vi "DAQ_Power.vi"(9 "stop":bool) -> ()   [LabVIEW 2020]
uses:
  <vilib>/Utility/error.llb/DialogType.ctl
  <vilib>/ULx/Create Channel.llb/ULx Create Channel (AI-Voltage-Basic).vi
  <vilib>/ULx/Timing.llb/ULx Timing (Sample Clock).vi
  <vilib>/ULx/Read.llb/ULx Read (Analog Wfm 1Chan NSamp).vi
panel:
  out "Power Graph":waveform(dbl)(graph)
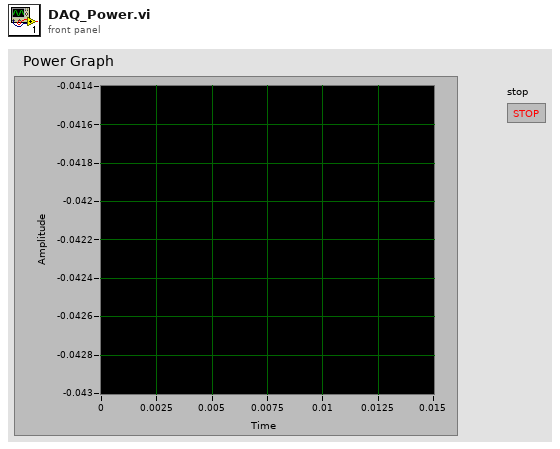
[diagram p1: front panel]
types:
  T1 = typedef "DialogType.ctl" = u16
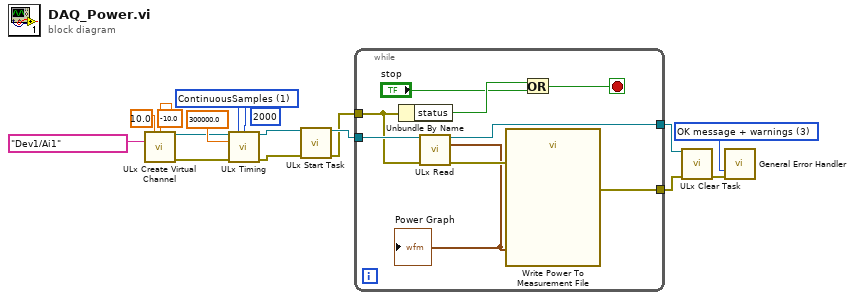
[diagram p0: block diagram]
diagram:
  w12 = 1 items=["FiniteSamples", "ContinuousSamples"] ("sample mode")
  w9 = T1 3 items=["no dialog", "OK message", "continue or stop message", "OK message + warnings", "continue/stop + warnings"] ("type of dialog (OK msg:1)")
  n1 = call-poly <vilib>:"ULx Create Virtual Channel.vi"("maximum value"=10.0, "minimum value"=-10.0, "physical channels"="Dev1/Ai1") -> ("task out"=w5:refnum<k24>, "error out"=w2:errorcluster)  [unwired: 11 in]
  n2 = call-poly <vilib>:"ULx Timing.vi"("task in"=w5, "sample mode"=w12, "samples per channel"=2000, "rate"=300000.0, "error in"=w2) -> ("task out"=w10:refnum<k24>, "error out"=w11:errorcluster)  [unwired: 9 in]
  n3 = call <vilib>:"ULx Start Task.vi"("task in"=w10, "error in"=w11) -> ("task out"=w6:refnum<k24>, "error out"=w3:errorcluster)  [unwired: 12 in]
  n4 = while {
    tunnel: w3 -> [w19]
    tunnel: w6 -> [w25]
    tunnel: [w24] -> w7
    tunnel: [w20] -> w8
    stop <- w22 stop-if-true
    n5 = Unbundle By Name(w19) -> ("status"=w23:bool)
    n6 = call-poly <vilib>:"ULx Read.vi"("task in"=w25, "error in"=w19) -> ("task out"=w24:refnum<k24>, "data"=w18:waveform(dbl), "error out"=w21:errorcluster)  [unwired: 11 in]
    "Power Graph" <- w18
    n7 = call "Write Power To Measurement File"("Signals"=w18, "error in (no error)"=w21) -> ("error out"=w20:errorcluster)  [unwired: 15 in, 2 out]
    n8 = Or(x=w23, y="stop") -> (x .or. y?=w22:bool)
  }
  n9 = call <vilib>:"ULx Clear Task.vi"("task in"=w7, "error in"=w8) -> ("error out"=w4:errorcluster)  [unwired: 13 in]
  n10 = call <vilib>:"General Error Handler.vi"("type of dialog (OK msg:1)"=w9, "error in (no error)"=w4) -> ()  [unwired: 9 in, 5 out]
